vi "TB3000_on_off.vi"(8 "error in":errorcluster, 10 "On/Off":bool, 11 "VISA resource name in":refnum<visa-resource-name>) -> (0 "error out":errorcluster, 3 "VISA resource name out":refnum<visa-resource-name>)   [LabVIEW 2021]
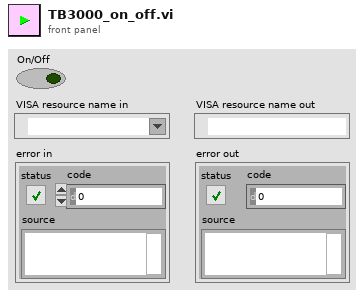
[diagram p1: front panel]
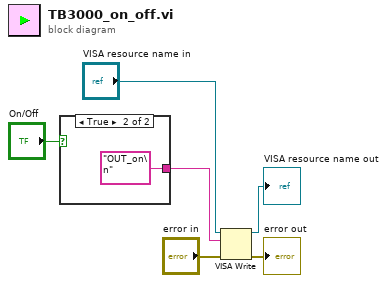
[diagram p0: block diagram]
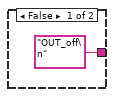
[diagram p2: hidden frame]
diagram:
  n1 = case shown="True" "On/Off" {
    tunnel: ["OUT_off\n" "OUT_on\n"] -> w2
    frame False {
    }
    frame True {
    }
  }
  n2 = VISA Write(VISA resource name="VISA resource name in", write buffer=w2, error in (no error)="error in") -> (VISA resource name out=→"VISA resource name out":refnum<visa-resource-name>, error out=→"error out":errorcluster)  [unwired: 1 out]
